vi "Scan.vi"() -> ()   [LabVIEW 2013]
uses:
  Tools/Line.ctl
panel:
  in  "Make":bool
  in  "Tab Control":enum32{"Template", "Array", "Output"}(tab)
  in  "Template":T1 caption="Template (array tag: MOD)"
  in  "Shuffle":bool
  in  "Build Array":bool
  out "Array":string[](array[string])
  in  "Step":dbl=0.1
  in  "Max":dbl=1.0
  in  "Min":dbl
  out "array size":i32
  in  "format string":string="%.4g"
  in  "SEQs":T1[](array[typedef])
  in  "Template":T1[](array[typedef])
  out "#":i32
  in  "Save":path
  in  "Stop Button":bool
  in  "Save Button":bool
  in  "Load Button":bool
  in  "New Button":bool
  # "Scan"
  # "Use an array to quickly create a sequence"
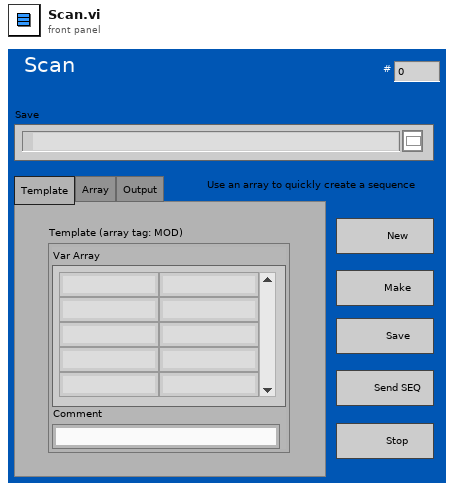
[diagram p1: front panel]
types:
  T1 = typedef "Line.ctl" = cluster{"Var Array":string[][], "Comment":string}
  T2 = enum16{"Left Button", "Center Button", "Right Button", "Window Close"}
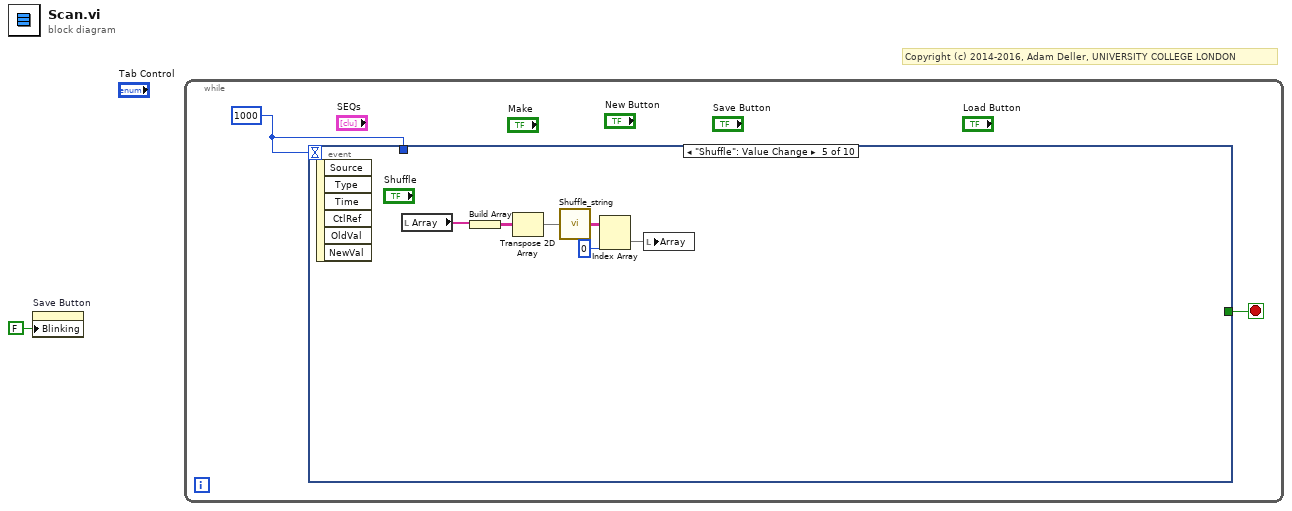
[diagram p0: block diagram]
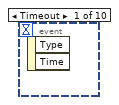
[diagram p2: hidden frame]
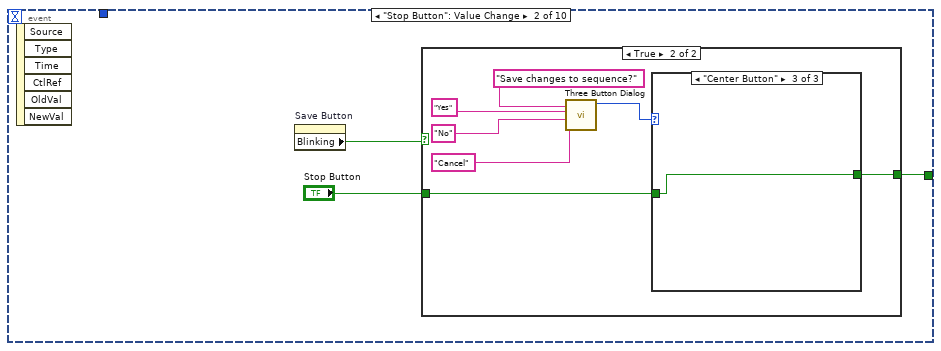
[diagram p3: hidden frame]
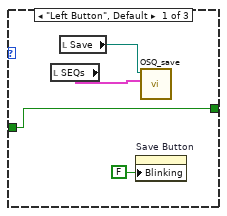
[diagram p5: hidden frame]
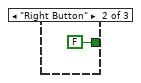
[diagram p6: hidden frame]
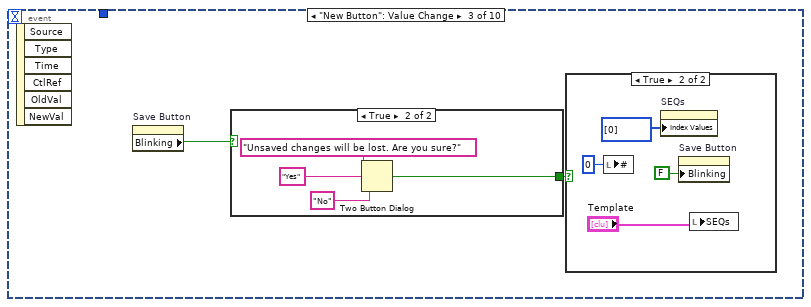
[diagram p7: hidden frame]
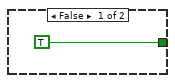
[diagram p9: hidden frame]
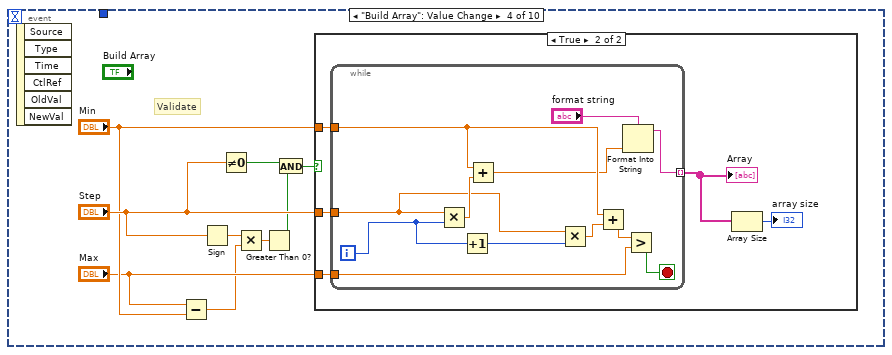
[diagram p10: hidden frame]
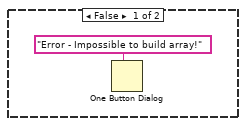
[diagram p11: hidden frame]
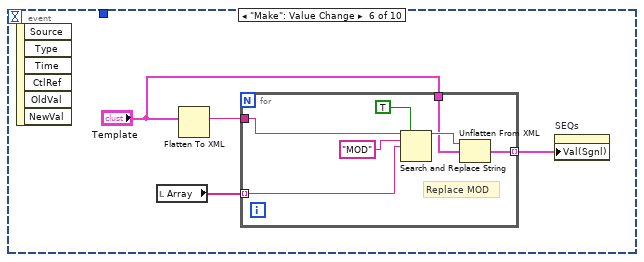
[diagram p12: hidden frame]
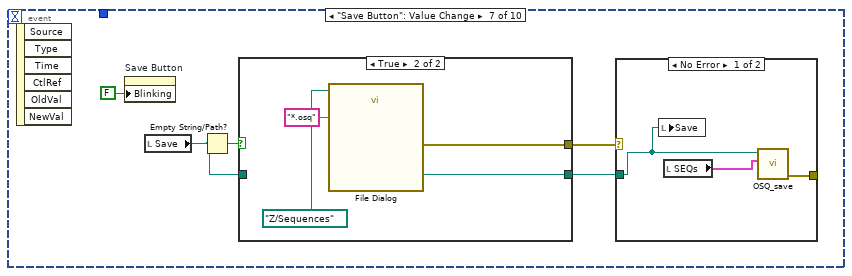
[diagram p13: hidden frame]
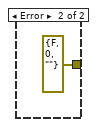
[diagram p14: hidden frame]
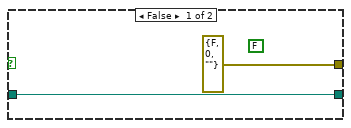
[diagram p15: hidden frame]
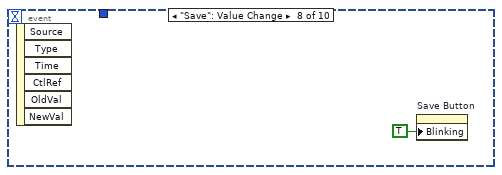
[diagram p16: hidden frame]
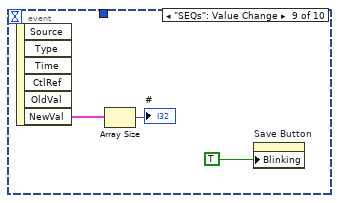
[diagram p17: hidden frame]
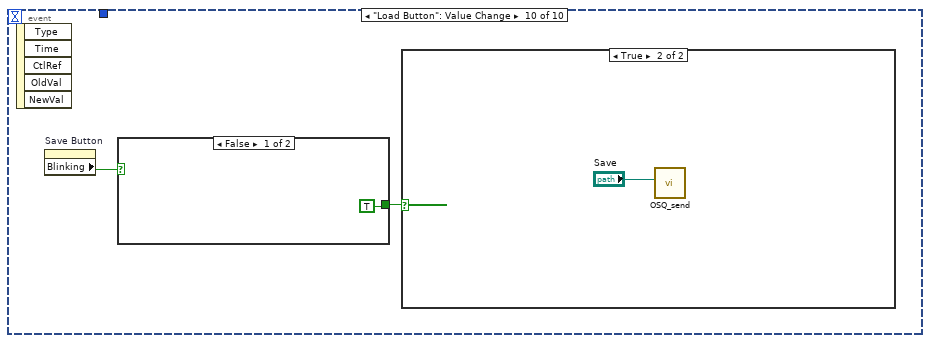
[diagram p18: hidden frame]
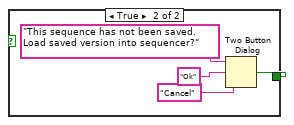
[diagram p20: hidden frame]
diagram:
  # "Copyright (c) 2014-2016, Adam Deller, UNIVERSITY COLLEGE LONDON"
  n1 = property on="Save Button" class="Bool"("Blinking"=FALSE) -> ()  [unwired: 2 in, 2 out]
  n2 = while {
    stop <- w3 stop-if-true
    w2 = 1000
    n3 = event shown="[4] \"Shuffle\": Value Change" {
      selector: _ -> [_ _ _ _ _ _ _ _ _ _]
      dyn-events: _ -> [_ _ _ _ _ _ _ _ _ _]
      timeout: w2 -> [_ _ _ _ _ _ _ _ _ _]
      tunnel: [_ w6 _ _ _ _ _ _ _ _] -> w3
      tunnel: w2 -> [_ _ _ _ _ _ _ _ _ _]
      event Timeout {
        n4 = event-data() -> ()  [unwired: 1 in, 2 out]
      }
      event "Stop Button": Value Change {
        n5 = event-data() -> ()  [unwired: 1 in, 6 out]
        n6 = property on="Save Button" class="Bool"() -> ("Blinking"=w5:bool)  [unwired: 2 in, 2 out]
        n7 = case shown="True" w5 {
          tunnel: [w7 w8] -> w6
          tunnel: "Stop Button" -> [w7 w9]
          frame False {
          }
          frame True {
            n8 = call <vilib>:"Three Button Dialog.vi"("Right Button Text (\"Cancel\")"="Cancel" ("Right Button Text (\"Cancel\")"), "Center Button Text (\"No\")"="No" ("F button name (\"Cancel\")"), "Left Button Text (\"Yes\")"="Yes" ("T button name (\"OK\")"), "message"="Save changes to sequence?") -> ("Which Button?"=w10:T2)  [unwired: 7 in]
            n9 = case shown="\"Center Button\"" w10 {
              tunnel: w9 -> [w18 _ w20]
              tunnel: [w18 FALSE ("Stop Button") w20] -> w8
              frame "Left Button", Default {
                n10 = local read "SEQs"() -> (w15:T1[])
                n11 = local read "Save"() -> (w17:path)
                n12 = property on="Save Button" class="Bool"("Blinking"=FALSE) -> ()  [unwired: 2 in, 2 out]
                n13 = call "OSQ_save.vi"("SEQs"=w15, "Save"=w17) -> ()  [unwired: 8 in, 2 out]
              }
              frame "Right Button" {
              }
              frame "Center Button" {
              }
            }
          }
        }
      }
      event "New Button": Value Change {
        n14 = event-data() -> ()  [unwired: 1 in, 6 out]
        n15 = property on="Save Button" class="Bool"() -> ("Blinking"=w21:bool)  [unwired: 2 in, 2 out]
        n16 = case shown="True" w21 {
          tunnel: [TRUE w28] -> w22
          frame False {
          }
          frame True {
            n17 = Two Button Dialog(message="Unsaved changes will be lost. Are you sure?", 1:"No" ("F button name (\"Cancel\")"), 2:"Yes" ("T button name (\"OK\")")) -> (T button?=w28:bool)
          }
        }
        n18 = case shown="True" w22 {
          frame False {
          }
          frame True {
            n19 = local write "#"(0 ("#")) -> ()
            n20 = property on="SEQs" class="Arr (strict)"("Index Values"=u32[] [0]) -> ()  [unwired: 2 in, 2 out]
            n21 = property on="Save Button" class="Bool"("Blinking"=FALSE) -> ()  [unwired: 2 in, 2 out]
            n22 = local write "SEQs"("Template") -> ()
          }
        }
      }
      event "Build Array": Value Change {
        # "Validate"
        n23 = event-data() -> ()  [unwired: 1 in, 6 out]
        n24 = Subtract(x="Max", y="Min") -> (x-y=w36:dbl)
        n25 = Sign(1:"Step") -> (0:w39:dbl)
        n26 = Not Equal To 0?(x="Step") -> (x != 0?=w33:bool)
        n27 = Multiply(x=w39, y=w36) -> (x*y=w35:dbl)
        n28 = Greater Than 0?(x=w35) -> (x > 0?=w32:bool)
        n29 = And(x=w33, y=w32) -> (x .and. y?=w34:bool)
        n30 = case shown="True" w34 {
          tunnel: "Min" -> [_ w46]
          tunnel: "Step" -> [_ w45]
          tunnel: "Max" -> [_ w44]
          frame False {
            n31 = One Button Dialog(message="Error - Impossible to build array!") -> ()  [unwired: 1 in, 1 out]
          }
          frame True {
            n32 = while {
              tunnel: w46 -> [w53]
              tunnel: [w47] -> w42 mode=indexing
              tunnel: w45 -> [w55]
              tunnel: w44 -> [w51]
              i -> [w57]
              stop <- w50 stop-if-true
              n33 = Multiply(x=w55, y=w57) -> (x*y=w58:dbl)
              n34 = Increment(x=w57) -> (x+1=w56:i32)
              n35 = Add(x=w53, y=w58) -> (x+y=w48:dbl)
              n36 = Multiply(x=w55, y=w56) -> (x*y=w54:dbl)
              n37 = Add(x=w53, y=w54) -> (x+y=w52:dbl)
              n38 = Format Into String(format string="format string", w48) -> (resulting string=w47:string)  [unwired: 2 in, 1 out]
              n39 = Greater?(x=w52, y=w51) -> (0:w50:bool)
            }
            "Array" <- w42
            n40 = Array Size(array=w42) -> (size(s)=→"array size":i32)
          }
        }
      }
      event "Shuffle": Value Change {
        n41 = event-data() -> ()  [unwired: 1 in, 6 out]
        n42 = local read "Array"() -> (w64:string[])
        n43 = Build Array(w64) -> (w61:string[][])
        n44 = Transpose 2D Array(2D array=w61) -> (transposed array=w60:string[][])
        n45 = call "Shuffle_string.vi"("Array IN"=w60) -> ("Array OUT"=w63:string[][])
        n46 = Index Array(array=w63, index (col)=0 ("disabled index (col)")) -> (element=w62:string[])  [unwired: 1 in]
        n47 = local write "Array"(w62) -> ()
      }
      event "Make": Value Change {
        n48 = event-data() -> ()  [unwired: 1 in, 6 out]
        n49 = local read "Array"() -> (w67:string[])
        n50 = Flatten To XML(anything="Template") -> (xml string=w68:string)
        n51 = for {
          tunnel: w68 -> [w74]
          tunnel: w67 -> [w69] mode=indexing
          tunnel: [w71] -> w65 mode=indexing
          tunnel: "Template" -> [w70]
          # "Replace MOD"
          n52 = Search and Replace String(replace all?=TRUE ("replace all? (F)"), input string=w74, search string="MOD", replace string=w69) -> (result string=w72:string)  [unwired: 4 in, 3 out]
          n53 = Unflatten From XML(xml string=w72, type=w70) -> (value=w71:T1)  [unwired: 1 in, 1 out]
        }
        n54 = property on="SEQs" class="Arr (strict)"("Val(Sgnl)"=w65) -> ()  [unwired: 2 in, 2 out]
      }
      event "Save Button": Value Change {
        n55 = event-data() -> ()  [unwired: 1 in, 6 out]
        n56 = property on="Save Button" class="Bool"("Blinking"=FALSE) -> ()  [unwired: 2 in, 2 out]
        n57 = local read "Save"() -> (w78:path)
        n58 = Empty String/Path?(string/path=w78) -> (empty?=w79:bool)
        n59 = case shown="True" w79 {
          tunnel: [w86 w90] -> w77
          tunnel: w78 -> [w86 _]
          tunnel: [errorcluster {"status"=FALSE, "code"=0, "source"=""} ("error out") w87] -> w76
          frame False {
            (unwired) FALSE ("cancelled")
          }
          frame True {
            n60 = call "File Dialog"("start path"=path "Z:/Sequences", "pattern (all files)"="*.osq") -> ("selected path"=w90:path, "error out"=w87:errorcluster)  [unwired: 10 in, 2 out]
          }
        }
        n61 = case shown="No Error" w76 {
          tunnel: w77 -> [w82 _]
          tunnel: [w81 errorcluster {"status"=FALSE, "code"=0, "source"=""} ("error out")] -> _
          frame No Error {
            n62 = local write "Save"(w82) -> ()
            n63 = local read "SEQs"() -> (w83:T1[])
            n64 = call "OSQ_save.vi"("SEQs"=w83, "Save"=w82) -> ("error out"=w81:errorcluster)  [unwired: 8 in, 1 out]
          }
          frame Error {
          }
        }
      }
      event "Save": Value Change {
        n65 = event-data() -> ()  [unwired: 1 in, 6 out]
        n66 = property on="Save Button" class="Bool"("Blinking"=TRUE) -> ()  [unwired: 2 in, 2 out]
      }
      event "SEQs": Value Change {
        n67 = event-data() -> ("NewVal"=w93:T1[])  [unwired: 1 in, 5 out]
        n68 = Array Size(array=w93) -> (size(s)=→"#":i32)
        n69 = property on="Save Button" class="Bool"("Blinking"=TRUE) -> ()  [unwired: 2 in, 2 out]
      }
      event "Load Button": Value Change {
        n70 = event-data() -> ()  [unwired: 1 in, 5 out]
        n71 = property on="Save Button" class="Bool"() -> ("Blinking"=w96:bool)  [unwired: 2 in, 2 out]
        n72 = case shown="False" w96 {
          tunnel: [TRUE w99] -> w95
          frame False {
          }
          frame True {
            n73 = Two Button Dialog(message="This sequence has not been saved.  Load saved version into sequencer?", 1:"Cancel" ("F button name (\"Cancel\")"), 2:"Ok" ("T button name (\"OK\")")) -> (T button?=w99:bool)
          }
        }
        n74 = case shown="True" w95 {
          frame False {
          }
          frame True {
            n75 = call "OSQ_send.vi"("Sequence File"="Save") -> ()  [unwired: 11 in]
          }
        }
      }
    }
  }
